vi "LakeShore 370.vi"(2 "Point #":i32, 3 "Parameters":dbl[](array[numeric]) format="%.3e", 4 "Instrument Address":refnum<visa-resource-name>) -> (0 "Stop":bool, 1 "Measurement":dbl[](array[numeric]) format="%.6e")   [LabVIEW 2020]
doc: "This VI reads a single reading from a LakeShore 370 Temperature Controller. The stop boolean is always false. If no reading is obtained a single zero is returned.\nParameter 0 - 0=Resistance, 1=Temperature, 2=Heater Power\nParameter 1 - Channel to read, channel 0 is scan channel\nScott Hannahs, <sth@magnet.fsu.edu> NHMFL-FSU, May 2003"
panel:
  # "The first parameter tells it\nHeater power if =2\nto read temperature if =1\nResistance if =0\nThe second is channel #"
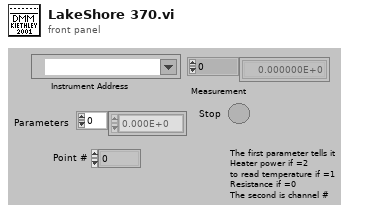
[diagram p1: front panel]
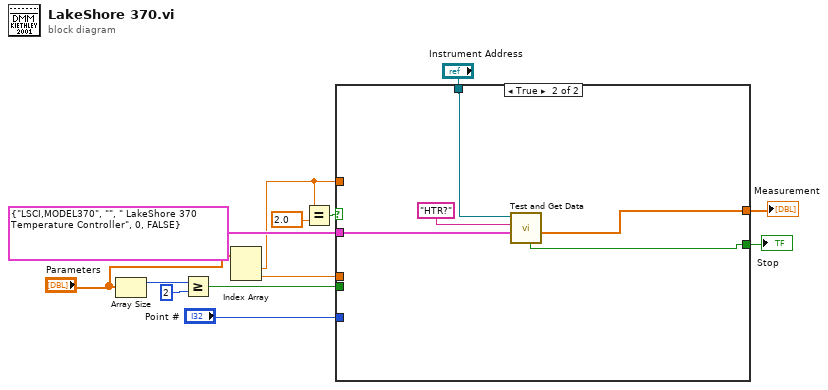
[diagram p0: block diagram]
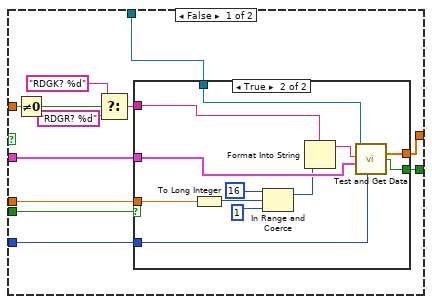
[diagram p2: hidden frame]
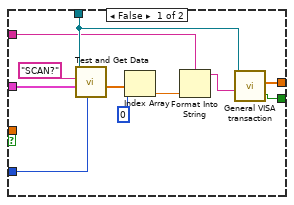
[diagram p3: hidden frame]
diagram:
  n1 = Array Size(array="Parameters") -> (size(s)=w7:i32)
  n2 = Greater Or Equal?(x=w7, y=2) -> (x >= y?=w10:bool)
  n3 = Index Array(array="Parameters") -> (element #1=w3:dbl, element #2=w5:dbl)  [unwired: 2 in]
  n4 = Equal?(x=w3, y=2.0) -> (x = y?=w4:bool)
  n5 = case shown="True" w4 {
    tunnel: cluster{string, string, string, u32, bool} {"LSCI,MODEL370", "", " LakeShore 370 Temperature Controller", 0, FALSE} -> [w25 w51]
    tunnel: [w24 w53] -> w12
    tunnel: [w23 w52] -> w11
    tunnel: w10 -> [w22 _]
    tunnel: "Point #" -> [w21 _]
    tunnel: w5 -> [w20 _]
    tunnel: w3 -> [w19 _]
    tunnel: "Instrument Address" -> [w14 w49]
    frame False {
      n6 = Not Equal To 0?(x=w19) -> (x != 0?=w18:bool)
      n7 = Select(t="RDGK? %d" ("Format String"), s=w18, f="RDGR? %d" ("Format String")) -> (s? t:f=w17:string)
      n8 = case shown="True" w22 {
        tunnel: w25 -> [w36 w45]
        tunnel: w14 -> [w31 w48]
        tunnel: [w30 w44] -> w24
        tunnel: [w29 w43] -> w23
        tunnel: w21 -> [w27 w47]
        tunnel: w20 -> [_ w38]
        tunnel: w17 -> [w26 w37]
        frame False {
          n9 = call "Test and Get Data.vi"("Point #"=w27, "Instrument Info"=w36, "Command String"="SCAN?", "VISA Sesson"=w31) -> ("Measurement"=w34:dbl[])  [unwired: 2 in, 4 out]
          n10 = Index Array(array=w34, index=0 ("Index")) -> (element=w32:dbl)
          n11 = Format Into String(format string=w26, w32) -> (resulting string=w28:string)  [unwired: 2 in, 1 out]
          n12 = call "General VISA transaction.vi"("Command String"=w28, "VISA Session"=w31) -> ("Measurement"=w30:dbl[], "Stop"=w29:bool)  [unwired: 4 in, 4 out]
        }
        frame True {
          n13 = To Long Integer(number=w38) -> (32bit integer=w39:i32)
          n14 = In Range and Coerce(upper limit=16, x=w39, lower limit=1) -> (coerced(x)=w42:i32)  [unwired: 1 out]
          n15 = Format Into String(format string=w37, w42) -> (resulting string=w46:string)  [unwired: 2 in, 1 out]
          n16 = call "Test and Get Data.vi"("Point #"=w47, "Instrument Info"=w45, "Command String"=w46, "VISA Sesson"=w48) -> ("Measurement"=w44:dbl[], "Stop"=w43:bool)  [unwired: 2 in, 3 out]
        }
      }
    }
    frame True {
      n17 = call "Test and Get Data.vi"("Instrument Info"=w51, "Command String"="HTR?", "VISA Sesson"=w49) -> ("Measurement"=w53:dbl[], "Stop"=w52:bool)  [unwired: 3 in, 3 out]
    }
  }
  "Stop" <- w11
  "Measurement" <- w12
